vi "ProcessStarted_Notification.vi"(8 "error in (no error)":errorcluster, 10 "This VI":refnum<vi>, 11 "DebuggingTerminal in":refnum<class "DebuggingTerminal.lvclass">) -> (0 "error out":errorcluster, 3 "DebuggingTerminal out":refnum<class "DebuggingTerminal.lvclass">)   [LabVIEW 2013, in "MQTT Base.lvlib" / "DebuggingTerminal.lvclass"]
uses:
  DebuggingTerminal.lvclass
  DebuggingTerminal.lvclass/DebuggingTerminal.ctl
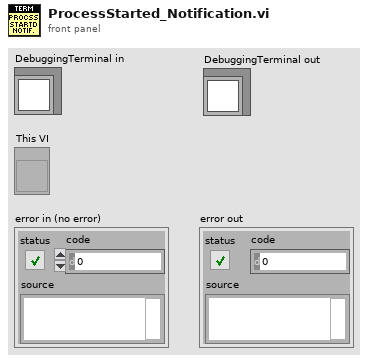
[diagram p1: front panel]
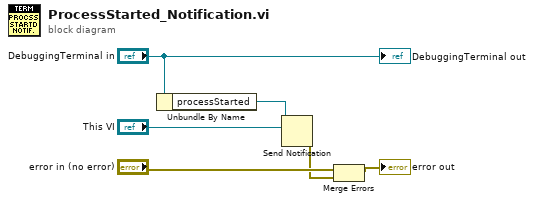
[diagram p0: block diagram]
diagram:
  n1 = Unbundle By Name("DebuggingTerminal in") -> ("processStarted"=w6:refnum<notifier>)
  n2 = Send Notification(notification="This VI", notifier=w6) -> (error out=w1:errorcluster)  [unwired: 1 in, 1 out]
  n3 = Merge Errors("error in (no error)", w1) -> (→"error out":errorcluster)
  "DebuggingTerminal out" <- "DebuggingTerminal in"
